vi "shared-dependency-sequential-test.vi"(8 "error in (no error)":errorcluster) -> (0 "error out":errorcluster)   [LabVIEW 2021]
uses:
  _test-support-SMOs/SMO.SelfTerminatingOverride/SMO.SelfTerminatingOverride.lvclass
  <vilib>/addons/_JKI Toolkits/Caraya/classes/Assert/Assert.lvclass
  <vilib>/addons/_JKI Toolkits/Caraya/classes/Test/Test.lvclass
  src/SMO/SMO.lvclass
  C:/Repositories/SMO/tests/_test-support-SMOs/SMO.SelfTerminating/SMO.SelfTerminating.lvclass
  C:/Repositories/SMO/src/SMO/SMO.lvclass
  C:/Repositories/SMO/tests/_test-support-SMOs/SMO.SelfTerminatingOverride/SMO.SelfTerminatingOverride.lvclass
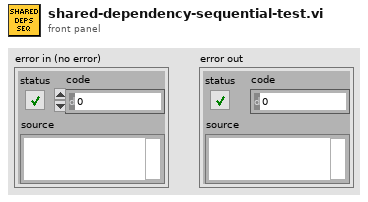
[diagram p1: front panel]
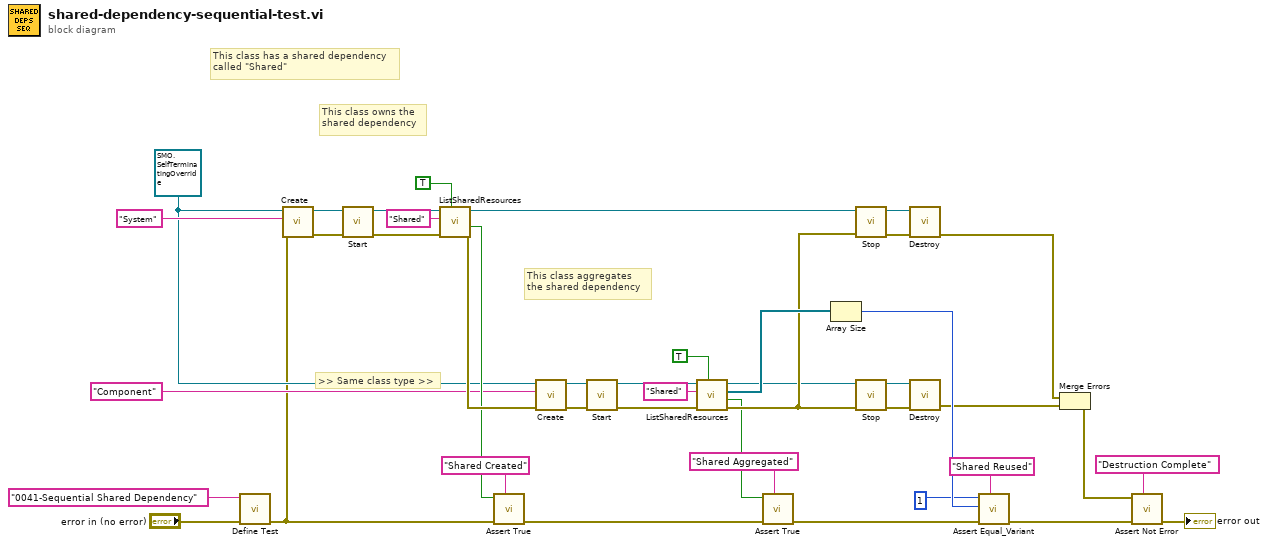
[diagram p0: block diagram]
diagram:
  w6 = refnum<class "SMO.SelfTerminatingOverride.lvclass"> refnum ("SMO.SelfTerminatingOverride.lvclass")
  # ">> Same class type >>"
  # "This class has a shared dependency\ncalled \"Shared\""
  # "This class aggregates\nthe shared dependency"
  # "This class owns the\nshared dependency"
  n1 = call <vilib>:"Define Test.vi"("error in (no error)"="error in (no error)", "Label (VI Title)"="0041-Sequential Shared Dependency") -> ("error out"=w3:errorcluster)  [unwired: 9 in]
  n2 = call "Create.vi"("error in (no error)"=w3, "Subsystem Name (optional)"="System", "SMO"=w6) -> ("error out"=w9:errorcluster, "SMO out"=w8:refnum<class "SMO.SelfTerminatingOverride.lvclass">)  [unwired: 6 in, 1 out]
  n3 = call "Start.vi"("error in (no error)"=w9, "SMO"=w8) -> ("error out"=w23:errorcluster, "SMO out"=w19:refnum<class "SMO.SelfTerminatingOverride.lvclass">)  [unwired: 8 in]
  n4 = call "ListSharedResources.vi"("exact name? (F: regex)"=TRUE, "error in (no error)"=w23, "Filter (regex|name)"="Shared", "SMO in"=w19) -> ("error out"=w24:errorcluster, "resources found?"=w21:bool, "SMO out"=w34:refnum<class "SMO.SelfTerminatingOverride.lvclass">)  [unwired: 4 in, 1 out]
  n5 = call <vilib>:"Assert True.vi"("Label"="Shared Created" ("Filter (regex|name)"), "error in (no error)"=w3, "True?"=w21) -> ("error out"=w30:errorcluster)  [unwired: 8 in]
  n6 = call "Create.vi"("error in (no error)"=w24, "Subsystem Name (optional)"="Component", "SMO"=w6) -> ("error out"=w14:errorcluster, "SMO out"=w13:refnum<class "SMO.SelfTerminatingOverride.lvclass">)  [unwired: 6 in, 1 out]
  n7 = call "Start.vi"("error in (no error)"=w14, "SMO"=w13) -> ("error out"=w28:errorcluster, "SMO out"=w27:refnum<class "SMO.SelfTerminatingOverride.lvclass">)  [unwired: 8 in]
  n8 = call "ListSharedResources.vi"("exact name? (F: regex)"=TRUE, "error in (no error)"=w28, "Filter (regex|name)"="Shared", "SMO in"=w27) -> ("error out"=w33:errorcluster, "resources found?"=w32:bool, "Shared Resources"=w38:refnum<class "SMO.lvclass">[], "SMO out"=w29:refnum<class "SMO.SelfTerminatingOverride.lvclass">)  [unwired: 4 in]
  n9 = call <vilib>:"Assert True.vi"("Label"="Shared Aggregated" ("Filter (regex|name)"), "error in (no error)"=w30, "True?"=w32) -> ("error out"=w39:errorcluster)  [unwired: 8 in]
  n10 = Array Size(array=w38) -> (size(s)=w41:i32)
  n11 = call "Stop.vi"("error in (no error)"=w33, "SMO"=w34) -> ("error out"=w12:errorcluster, "SMO out"=w11:refnum<class "SMO.SelfTerminatingOverride.lvclass">)  [unwired: 8 in]
  n12 = call "Stop.vi"("error in (no error)"=w33, "SMO"=w29) -> ("error out"=w15:errorcluster, "SMO out"=w16:refnum<class "SMO.SelfTerminatingOverride.lvclass">)  [unwired: 8 in]
  n13 = call "Destroy.vi"("error in (no error)"=w12, "SMO"=w11) -> ("error out"=w18:errorcluster)  [unwired: 9 in]
  n14 = call "Destroy.vi"("error in (no error)"=w15, "SMO"=w16) -> ("error out"=w17:errorcluster)  [unwired: 9 in]
  n15 = call <vilib>:"Assert Equal_Variant.vi"("Label"="Shared Reused" ("Filter (regex|name)"), "error in (no error)"=w39, "Y"=w41, "X"=1) -> ("error out"=w40:errorcluster)  [unwired: 7 in]
  n16 = Merge Errors(w18, w17) -> (w36:errorcluster)
  n17 = call <vilib>:"Assert Not Error.vi"("Label"="Destruction Complete", "error in (no error)"=w40, "Not Error?"=w36) -> ("error out"=→"error out":errorcluster)  [unwired: 8 in]
